vi "Tracking v2.vi"(4 "Offset Home 2 RCM":dbl[](array[numeric])=[0.0, 0.0, 0.0, 0.0], 5 "Trajectory Cluster":T1, 6 "PID Cluster":T4={"L1 to L4 PID Cluster"={"L1 PID Gains"={"Kp"=0.005, "Kd"=0.5, "Ki"=0.0005}, "L2 PID Gains"={"Kp"=0.01, "Kd"=1.0, "Ki"=0.005}, "L3 PID Gains"={"Kp"=0.05, "Kd"=1.0, "Ki"=0.0005}, "L4 PID Gains"={"Kp"=0.1, "Kd"=0.1, "Ki"=0.0005}}, "Stage PID Cluster"={"Stage Z PID"={"Kp"=0.0005, "Kd"=0.001, "Ki"=0.0}, "Stage Y PID"={"Kp"=0.0003, "Kd"=0.01, "Ki"=0.0}, "Stage X PID"={"Kp"=0.0003, "Kd"=0.01, "Ki"=0.0}}, "OCT Z PID Gains"={"Kp"=0.0003, "Kd"=0.0001, "Ki"=0.01}}, 7 "No. Cycles":u8=1, 8 "error in":errorcluster, 10 "Prev Posit Cluster":T3={"Prev L1 to L4 Posit"=[-0.5319, -0.035669172703475985, -2.0566170657346783, 0.9099264705882353], "Prev Stage Posit"=[6.002553885707208, 5.996566124542428, 5.995469940427586], "Prev OCT Z Posit"=-0.0}, 11 "FPGA VI Reference In":refnum<k20>) -> (0 "error out":errorcluster, 2 "Last Posit Cluster":T2={"Last L1 to L4 Posit"=[0.0, 0.0, 0.0, 0.0], "Last Stage Posit"=[6.0, 6.0, 6.0], "Last OCT Z Posit"=0.0}, 3 "FPGA VI Reference Out":refnum<k20>)   [LabVIEW 2016]
uses:
  <vilib>/Platform/TimedLoop/XDataNode/timing_clust.ctl
  <vilib>/Platform/TimedLoop/XDataNode/nitl_modes.ctl
  <vilib>/Platform/TimedLoop/XDataNode/wakeup.ctl
  Global Variables.vi
  <vilib>/platform/TimedLoop/XDataNode/XDataNode.xnode
  <vilib>/Platform/TimedLoop/XDataNode/XDNodeRunTimeDep.lvlib
  Library/KevinLibraryAll/labview/KevLib01.lvlib
panel:
  out "In Servo Loop":bool
  out "Loading Finished":bool
  # "e"
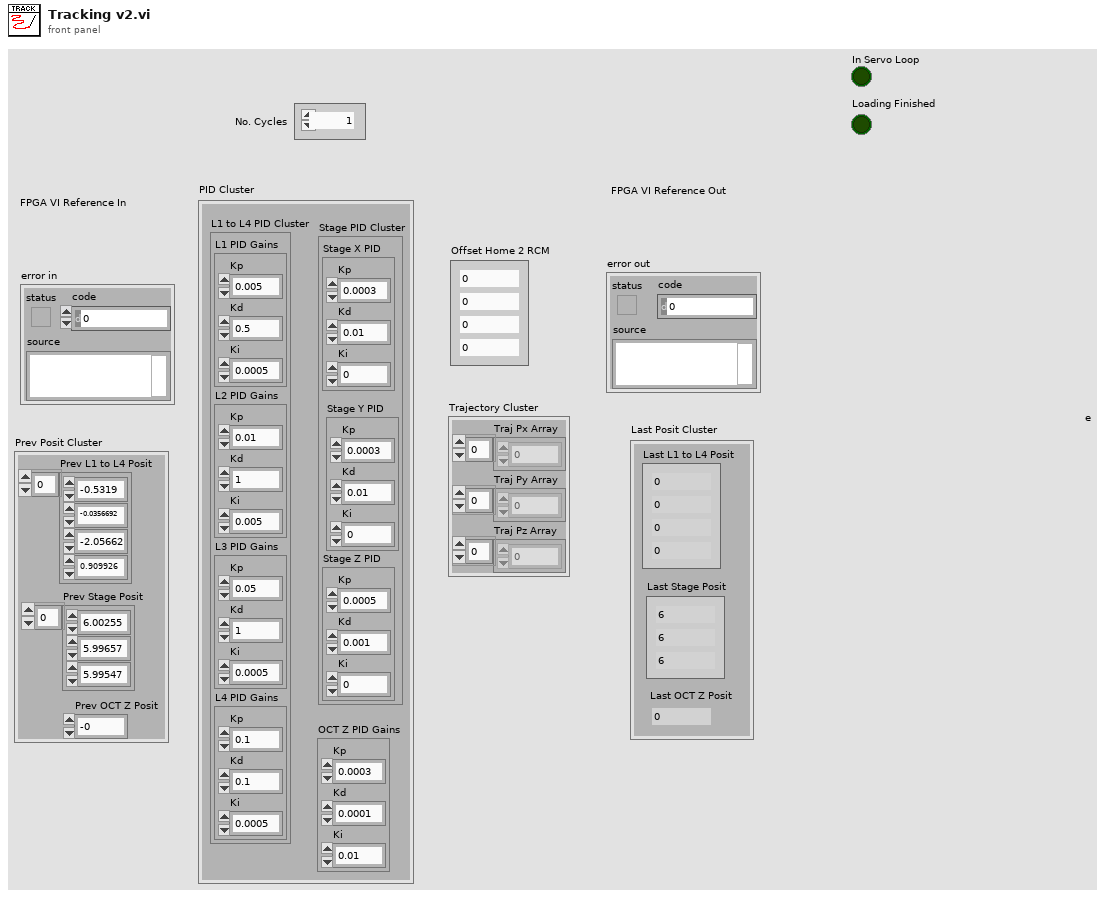
[diagram p1: front panel]
types:
  T1 = cluster{"Traj Px Array":dbl[], "Traj Py Array":dbl[], "Traj Pz Array":dbl[]}
  T2 = cluster{"Last L1 to L4 Posit":dbl[], "Last Stage Posit":dbl[], "Last OCT Z Posit":dbl}
  T3 = cluster{"Prev L1 to L4 Posit":dbl[], "Prev Stage Posit":dbl[], "Prev OCT Z Posit":dbl}
  T4 = cluster{"L1 to L4 PID Cluster":cluster{"L1 PID Gains":cluster{"Kp":dbl, "Kd":dbl, "Ki":dbl}, "L2 PID Gains":cluster{"Kp":dbl, "Kd":dbl, "Ki":dbl}, "L3 PID Gains":cluster{"Kp":dbl, "Kd":dbl, "Ki":dbl}, "L4 PID Gains":cluster{"Kp":dbl, "Kd":dbl, "Ki":dbl}}, "Stage PID Cluster":cluster{"Stage Z PID":cluster{"Kp":dbl, "Kd":dbl, "Ki":dbl}, "Stage Y PID":cluster{"Kp":dbl, "Kd":dbl, "Ki":dbl}, "Stage X PID":cluster{"Kp":dbl, "Kd":dbl, "Ki":dbl}}, "OCT Z PID Gains":cluster{"Kp":dbl, "Kd":dbl, "Ki":dbl}}
  T5 = typedef "XDNodeRunTimeDep.lvlib/timing_clust.ctl" = cluster{"Expected End [f-1]":u64, "Actual End [f-1]":u64, "Finished Late? [f-1]":bool, "Expected End [i-1]":u64, "Actual End [i-1]":u64, "Finished Late? [i-1]":bool, "Expected Start [i]":u64, "Actual Start [i]":u64, "Expected Start [f]":u64, "Actual Start [f]":u64, "Source Name":string, "Structure Name":string, "Period":i64, "Deadline":i64, "Offset":i64, "Start":i64, "Priority":i32, "Timeout":i32, "Mode":T6, "Wakeup Reason":T7, "Error":errorcluster, "Source Type":string, "Secondary Source Type":string, "Global End Time":u64, "Global Start Time":u64, "Frame Duration":u64, "Iteration Duration":u64, "Assigned CPU":i32, "I/O Scan Engine Mode":u32}
  T6 = typedef "XDNodeRunTimeDep.lvlib/nitl_modes.ctl" = enum32{"No Change", "Process missed periods, maintain original phase", "Discard missed periods, maintain original phase", "Process missed periods, ignore original phase", "Discard missed periods, ignore original phase"}
  T7 = typedef "XDNodeRunTimeDep.lvlib/wakeup.ctl" = enum32{"Normal", "Aborted", "Asynchronous wakeup", "Timing source error", "Timed loop error", "Timeout"}
  T8 = cluster{"L1 PID Gains":cluster{"Kp":dbl, "Kd":dbl, "Ki":dbl}, "L2 PID Gains":cluster{"Kp":dbl, "Kd":dbl, "Ki":dbl}, "L3 PID Gains":cluster{"Kp":dbl, "Kd":dbl, "Ki":dbl}, "L4 PID Gains":cluster{"Kp":dbl, "Kd":dbl, "Ki":dbl}}
  T9 = cluster{"Stage Z PID":cluster{"Kp":dbl, "Kd":dbl, "Ki":dbl}, "Stage Y PID":cluster{"Kp":dbl, "Kd":dbl, "Ki":dbl}, "Stage X PID":cluster{"Kp":dbl, "Kd":dbl, "Ki":dbl}}
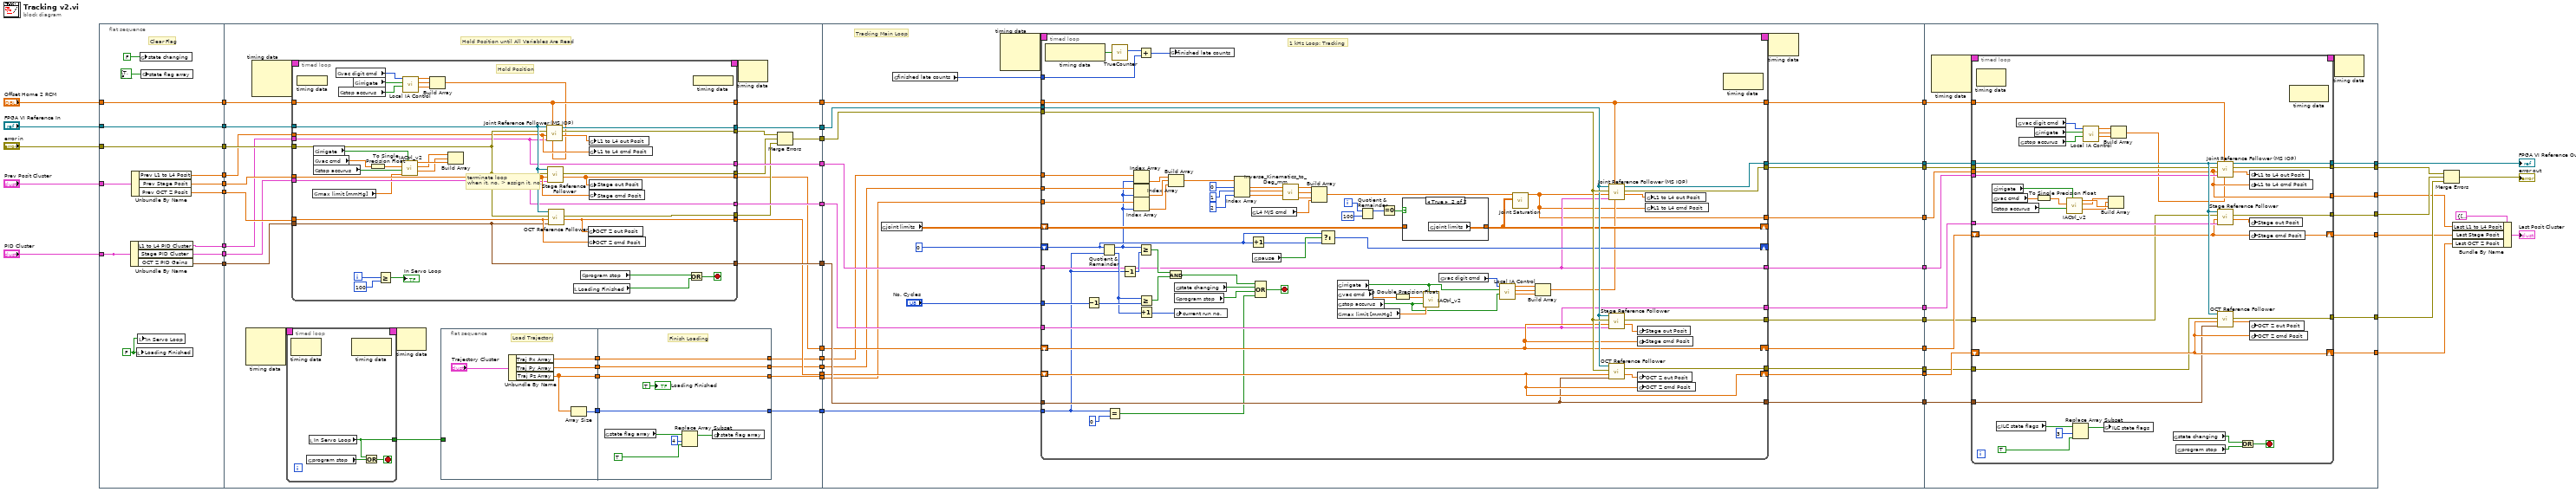
[diagram p0: block diagram]
diagram:
  n1 = flat-sequence {
    tunnel: [w59] -> w47
    tunnel: "FPGA VI Reference In" -> [w59]
    tunnel: "error in" -> [w58]
    tunnel: [w58] -> w44
    tunnel: "Prev Posit Cluster" -> [w57]
    tunnel: [w56] -> _
    tunnel: "PID Cluster" -> [w56]
    tunnel: [w55] -> w41
    tunnel: [w54] -> w40
    tunnel: [w53] -> w39
    tunnel: [w52] -> w38
    tunnel: [w51] -> w37
    tunnel: "Offset Home 2 RCM" -> [w51]
    tunnel: [w50] -> w32
    tunnel: [w48] -> w23
    tunnel: w47 -> [w94]
    tunnel: w44 -> [w93]
    tunnel: w41 -> [w92]
    tunnel: w40 -> [w91]
    tunnel: w39 -> [w90]
    tunnel: w38 -> [w89]
    tunnel: w37 -> [w88]
    tunnel: [w87] -> w35
    tunnel: [w86] -> w34
    tunnel: [w85] -> w33
    tunnel: w32 -> [w84]
    tunnel: [w83] -> w31
    tunnel: [w82] -> w30
    tunnel: [w81] -> w29
    tunnel: w23 -> [w80]
    tunnel: [w74] -> w22
    tunnel: [w73] -> w21
    tunnel: [w66] -> w20
    tunnel: [w65] -> w19
    tunnel: [w64] -> w18
    tunnel: [w62] -> w17
    tunnel: w35 -> [w183]
    tunnel: w34 -> [w168]
    tunnel: w33 -> [w182]
    tunnel: w31 -> [w180]
    tunnel: w30 -> [w179]
    tunnel: w29 -> [w178]
    tunnel: w22 -> [w170]
    tunnel: w21 -> [w169]
    tunnel: w20 -> [w167]
    tunnel: w19 -> [w166]
    tunnel: w18 -> [w165]
    tunnel: w17 -> [w157]
    tunnel: [w177] -> w16
    tunnel: [w176] -> w15
    tunnel: [w175] -> w14
    tunnel: [w174] -> w13
    tunnel: [w173] -> w12
    tunnel: [w172] -> w11
    tunnel: [w171] -> w10
    tunnel: [w161] -> w9
    tunnel: [w160] -> w8
    tunnel: [w159] -> w7
    tunnel: [w158] -> w6
    tunnel: [w275] -> w24
    tunnel: [w281] -> w2
    tunnel: [w276] -> w3
    tunnel: [w268] -> w5
    tunnel: [w269] -> w25
    tunnel: w16 -> [w273]
    tunnel: w15 -> [w272]
    tunnel: w14 -> [w277]
    tunnel: w13 -> [w279]
    tunnel: w12 -> [w282]
    tunnel: w11 -> [w278]
    tunnel: w10 -> [w280]
    tunnel: w9 -> [w283]
    tunnel: w8 -> [w274]
    tunnel: w7 -> [w271]
    tunnel: w6 -> [w270]
    tunnel: [w267] -> w4
    tunnel: [w266] -> w1
    frame #0 {
      w49 = FALSE ("Loading Finished")
      # "Clear Flag"
      n2 = Unbundle By Name(w56) -> ("L1 to L4 PID Cluster"=w52:T8, "Stage PID Cluster"=w50:T9, "OCT Z PID Gains"=w55:cluster{"Kp":dbl, "Kd":dbl, "Ki":dbl})
      n3 = Unbundle By Name(w57) -> ("Prev L1 to L4 Posit"=w48:dbl[], "Prev Stage Posit"=w54:dbl[], "Prev OCT Z Posit"=w53:dbl)
      n4 = local write "Loading Finished"(w49) -> ()
      n5 = local write "In Servo Loop"(w49) -> ()
      n6 = global write "Global Variables.vi" "state changing"(FALSE ("state changing")) -> ()
      n7 = global write "Global Variables.vi" "state flag array"(bool[] [TRUE, FALSE, FALSE, FALSE, FALSE, FALSE, FALSE, FALSE, FALSE] ("state flag array")) -> ()
    }
    frame #1 {
      # "terminate loop\nwhen it. no. > assign it. no."
      # "Hold Position until All Variables Are Read"
      n8 = node-c288() -> (w72:T5)  [unwired: 3 in]
      n9 = node-c288() -> (w79:T5)  [unwired: 3 in]
      n10 = timed-loop {
        timing: w72 -> [_]
        timing-out: [_] -> w71
        tunnel: [w109] -> w70
        stop <- w111 stop-if-true
        n11 = node-c288() -> ()  [unwired: 1 in, 1 out]
        n12 = global read "Global Variables.vi" "program stop"() -> (w110:bool)
        n13 = local read "In Servo Loop"() -> (w109:bool)
        n14 = node-c288() -> ()  [unwired: 1 in, 1 out]
        n15 = Or(x=w109, y=w110) -> (x .or. y?=w111:bool)
      }
      n16 = timed-loop {
        timing: w79 -> [_]
        timing-out: [_] -> w78
        tunnel: [w148] -> w74
        tunnel: [w147] -> w73
        tunnel: [w146] -> w87
        tunnel: [w145] -> w77
        tunnel: [w144] -> w76
        tunnel: [w143] -> w75
        tunnel: w94 -> [w142]
        tunnel: w93 -> [w141]
        tunnel: w92 -> [w136]
        tunnel: w80 -> [w139]
        tunnel: w91 -> [w140]
        tunnel: w90 -> [w138]
        tunnel: w89 -> [w134]
        tunnel: w88 -> [w137]
        tunnel: [w137] -> w86
        tunnel: w84 -> [w135]
        tunnel: [w136] -> w81
        tunnel: [w135] -> w82
        tunnel: [w134] -> w83
        i -> [w133]
        stop <- w152 stop-if-true
        # "Hold Position"
        n17 = node-c288 ("Output Node")() -> ()  [unwired: 1 in]
        n18 = global read "Global Variables.vi" "max limit [mmHg]"() -> (w123:dbl)
        n19 = global read "Global Variables.vi" "irrigate"() -> (w129:bool)
        n20 = global read "Global Variables.vi" "vac cmd"() -> (w126:sgl)
        n21 = global read "Global Variables.vi" "stop accurus"() -> (w125:bool)
        n22 = global read "Global Variables.vi" "vac digit cmd"() -> (w121:i8)
        n23 = global read "Global Variables.vi" "stop accurus"() -> (w120:bool)
        n24 = global read "Global Variables.vi" "irrigate"() -> (w122:bool)
        n25 = To Single Precision Float(number=w126) -> (single precision float=w127:sgl)
        n26 = Greater Or Equal?(x=w133, y=100) -> (x >= y?=→"In Servo Loop":bool)
        n27 = call "IACtrl_v2.vi"("Irrigate?"=w129, "Max Limit [mmHg]"=w123, "E-Stop Vacuum"=w125, "Vacuum Force [mmHg]"=w127) -> ("Accurus ChB Vout"=w124:dbl, "Accurus ChA Vout"=w128:dbl, "Accurus Engaged Vout"=w130:dbl)  [unwired: 4 in, 1 out]
        n28 = call "Local IA Control.vi"("E-Stop Vacuum"=w120, "Irrigate?"=w122, "8bit integer"=w121) -> ("Accurus Engaged Vout"=w117:dbl, "Accurus ChB Vout"=w118:dbl, "Accurus ChA Vout"=w119:dbl)  [unwired: 6 in]
        n29 = Build Array(w119, w118, w117) -> (w116:dbl[])
        n30 = Build Array(w128, w124, w130) -> ()  [unwired: 1 out]
        n31 = call "Joint Reference Follower (MS IOP).vi"("Acc Ctrl Array"=w116, "Offset Home2RCM [deg/mm]"=w137, "PID Ctrl Cluster"=w134, "Ref Array [deg/mm]"=w139, "error in"=w141, "FPGA VI Reference In"=w142) -> ("Output Posit Array [deg/mm]"=w149:dbl[], "error out"=w145:errorcluster, "FPGA VI Reference Out"=w146:refnum<k20>)  [unwired: 3 in]
        n32 = call "Stage Reference Follower.vi"("Stage PID Cluster"=w135, "Stage cmd Posit [mm]"=w140, "error in"=w141, "FPGA VI Reference In"=w142) -> ("Stage out Posit [mm]"=w148:dbl[], "error out"=w144:errorcluster)  [unwired: 5 in, 1 out]
        n33 = call "OCT Reference Follower.vi"("OCT Z PID Gains"=w136, "OCT  Z cmd Posit [mm]"=w138, "error in"=w141, "FPGA VI Reference In"=w142) -> ("OCT  Z out Posit [mm]"=w147:dbl, "error out"=w143:errorcluster)  [unwired: 5 in, 1 out]
        n34 = local read "Loading Finished"() -> (w151:bool)
        n35 = global read "Global Variables.vi" "program stop"() -> (w150:bool)
        n36 = global write "Global Variables.vi" "OCT Z out Posit"(w147) -> ()
        n37 = global write "Global Variables.vi" "OCT Z cmd Posit"(w138) -> ()
        n38 = global write "Global Variables.vi" "L1 to L4 out Posit"(w149) -> ()
        n39 = global write "Global Variables.vi" "L1 to L4 cmd Posit"(w139) -> ()
        n40 = global write "Global Variables.vi" "Stage out Posit"(w148) -> ()
        n41 = global write "Global Variables.vi" "Stage cmd Posit"(w140) -> ()
        n42 = Or(x=w150, y=w151) -> (x .or. y?=w152:bool)
        n43 = node-c288() -> ()  [unwired: 1 out]
      }
      n44 = node-c288(w71) -> ()  [unwired: 1 out]
      n45 = flat-sequence {
        tunnel: w70 -> [_]
        tunnel: [w98] -> w69
        tunnel: [w97] -> w68
        tunnel: [w96] -> w67
        tunnel: [w95] -> w63
        tunnel: w69 -> [w105]
        tunnel: w68 -> [w106]
        tunnel: w67 -> [w107]
        tunnel: [w107] -> w66
        tunnel: [w106] -> w65
        tunnel: [w105] -> w64
        tunnel: w63 -> [w104]
        tunnel: [w104] -> w62
        frame #0 {
          # "Load Trajectory"
          n46 = Unbundle By Name("Trajectory Cluster") -> ("Traj Px Array"=w96:dbl[], "Traj Py Array"=w97:dbl[], "Traj Pz Array"=w98:dbl[])
          n47 = Array Size(array=w98) -> (size(s)=w95:i32)
        }
        frame #1 {
          # "Finish Loading"
          n48 = global read "Global Variables.vi" "state flag array"() -> (w101:bool[])
          n49 = Replace Array Subset(array=w101, new element=TRUE ("new element/subarray"), index=4) -> (w100:bool[])
          n50 = global write "Global Variables.vi" "state flag array"(w100) -> ()
          "Loading Finished" <- TRUE ("Loading Finished")
        }
      }
      n51 = node-c288(w78) -> ()  [unwired: 1 out]
      n52 = Merge Errors(w77, w76, w75) -> (w85:errorcluster)
    }
    frame #2 {
      # "Tracking Main Loop"
      n53 = global read "Global Variables.vi" "joint limits"() -> (w162:dbl[][])
      n54 = global read "Global Variables.vi" "finished late counts"() -> (w181:u16)
      n55 = node-c288() -> (w185:T5)  [unwired: 3 in]
      n56 = timed-loop {
        timing: w185 -> [_]
        timing-out: [_] -> w184
        tunnel: w167 -> [w258]
        tunnel: w166 -> [w257]
        tunnel: w165 -> [w241]
        tunnel: w183 -> [w253]
        tunnel: w168 -> [w202]
        tunnel: w182 -> [w254]
        tunnel: [w255] -> w177
        tunnel: w180 -> [w199]
        tunnel: w181 -> [w249]
        tunnel: w179 -> [w201]
        tunnel: w178 -> [w200]
        shift-right: [w204] -> w172
        shift-left: w170 -> [w204]
        shift-right: [w203] -> w171
        shift-left: w169 -> [w203]
        tunnel: [w246] -> w175
        tunnel: [w245] -> w174
        tunnel: [w244] -> w176
        tunnel: [w194] -> w173
        tunnel: "No. Cycles" -> [w217]
        shift-right: [w215] -> _
        shift-left: 0 ("No. Cycles") -> [w198]
        tunnel: w157 -> [w197]
        shift-right: [w210] -> _
        shift-left: w162 -> [w209]
        tunnel: [w202] -> w161
        tunnel: [w201] -> w158
        tunnel: [w200] -> w160
        tunnel: [w199] -> w159
        i -> [w214]
        stop <- w222 stop-if-true
        # "Hold Position if not Engaged"
        # "1 kHz Loop: Tracking"
        n57 = node-c288() -> (w252:bool)  [unwired: 1 in]
        n58 = Decrement(x=w217) -> (x-1=w228:u8)
        n59 = Quotient & Remainder(x=w198, y=w197) -> (x-y*floor(x/y)=w192:i32, floor(x/y)=w216:i32)
        n60 = Equal?(x=w197, y=0) -> (x = y?=w195:bool)
        n61 = call "TrueCounter.vi"("True?"=w252) -> ("True Count"=w250:u16)  [unwired: 10 in]
        n62 = Decrement(x=w197) -> (x-1=w229:i32)
        n63 = Index Array(array=w258, index=w192) -> (element=w233:dbl)
        n64 = Index Array(array=w257, index=w192) -> (element=w232:dbl)
        n65 = Index Array(array=w241, index=w192) -> (element=w231:dbl)
        n66 = Add(x=w250, y=w249) -> (x+y=w251:u16)
        n67 = Greater Or Equal?(x=w192, y=w229) -> (x >= y?=w227:bool)
        n68 = Greater Or Equal?(x=w216, y=w228) -> (x >= y?=w226:bool)
        n69 = Increment(x=w216) -> (x+1=w218:i32)
        n70 = And(x=w227, y=w226) -> (x .and. y?=w225:bool)
        n71 = Build Array(w233, w232, w231) -> (w230:dbl[])
        n72 = global write "Global Variables.vi" "finished late counts"(w251) -> ()
        n73 = global read "Global Variables.vi" "state changing"() -> (w224:bool)
        n74 = global read "Global Variables.vi" "program stop"() -> (w223:bool)
        n75 = global write "Global Variables.vi" "current run no."(w218) -> ()
        n76 = Index Array(array=w230, index #1=0 ("index"), index #2=1 ("index"), index #3=2 ("index")) -> (element #1=w236:dbl, element #2=w235:dbl, element #3=w234:dbl)
        n77 = Increment(x=w198) -> (x+1=w219:i32)
        n78 = global read "Global Variables.vi" "L4 M/S cmd"() -> (w221:dbl)
        n79 = global read "Global Variables.vi" "pause"() -> (w220:bool)
        n80 = Compound Arithmetic op=OR(w225, w224, w223, w195) -> (w222:bool)
        n81 = call "Inverse_Kinematics_to_Deg_mm.vi"("pz"=w234, "py"=w235, "px"=w236) -> ("L3 [mm]"=w242:dbl, "L2 [deg]"=w243:dbl, "L1 [deg]"=w256:dbl)
        n82 = Build Array(w256, w243, w242, w221) -> (w240:dbl[])
        n83 = Select(t=w198, s=w220, f=w219) -> (s? t:f=w215:i32)
        n84 = global read "Global Variables.vi" "irrigate"() -> (w189:bool)
        n85 = global read "Global Variables.vi" "vac cmd"() -> (w208:sgl)
        n86 = global read "Global Variables.vi" "stop accurus"() -> (w188:bool)
        n87 = global read "Global Variables.vi" "max limit [mmHg]"() -> (w206:dbl)
        n88 = Quotient & Remainder(x=w214, y=100) -> (x-y*floor(x/y)=w212:i32)  [unwired: 1 out]
        n89 = Equal To 0?(x=w212) -> (x = 0?=w211:bool)
        n90 = To Double Precision Float(number=w208) -> (double precision float=w207:dbl)
        n91 = case shown="True" w211 {
          tunnel: [w259 w260] -> w210
          tunnel: w209 -> [w259 _]
          frame False {
          }
          frame True {
            n92 = global read "Global Variables.vi" "joint limits"() -> (w260:dbl[][])
          }
        }
        n93 = call "IACtrl_v2.vi"("Irrigate?"=w189, "Max Limit [mmHg]"=w206, "E-Stop Vacuum"=w188, "Vacuum Force [mmHg]"=w207) -> ()  [unwired: 4 in, 4 out]
        n94 = global read "Global Variables.vi" "vac digit cmd"() -> (w190:i8)
        n95 = call "Local IA Control.vi"("E-Stop Vacuum"=w188, "Irrigate?"=w189, "8bit integer"=w190) -> ("Accurus Engaged Vout"=w186:dbl, "Accurus ChB Vout"=w187:dbl, "Accurus ChA Vout"=w191:dbl)  [unwired: 6 in]
        n96 = call "Joint Saturation.vi"("Joint Bounds [Deg/mm]"=w210, "Ref Array [Deg/mm]"=w240) -> ("Sat Ref Array [Deg/mm]"=w194:dbl[])  [unwired: 9 in]
        n97 = Build Array(w191, w187, w186) -> (w205:dbl[])
        n98 = call "Joint Reference Follower (MS IOP).vi"("Acc Ctrl Array"=w205, "Offset Home2RCM [deg/mm]"=w202, "PID Ctrl Cluster"=w199, "Ref Array [deg/mm]"=w194, "error in"=w254, "FPGA VI Reference In"=w253) -> ("Output Posit Array [deg/mm]"=w193:dbl[], "error out"=w244:errorcluster, "FPGA VI Reference Out"=w255:refnum<k20>)  [unwired: 3 in]
        n99 = call "Stage Reference Follower.vi"("Stage PID Cluster"=w201, "Stage cmd Posit [mm]"=w204, "error in"=w254, "FPGA VI Reference In"=w253) -> ("Stage out Posit [mm]"=w248:dbl[], "error out"=w246:errorcluster)  [unwired: 5 in, 1 out]
        n100 = call "OCT Reference Follower.vi"("OCT Z PID Gains"=w200, "OCT  Z cmd Posit [mm]"=w203, "error in"=w254, "FPGA VI Reference In"=w253) -> ("OCT  Z out Posit [mm]"=w247:dbl, "error out"=w245:errorcluster)  [unwired: 5 in, 1 out]
        n101 = global write "Global Variables.vi" "Stage out Posit"(w248) -> ()
        n102 = global write "Global Variables.vi" "Stage cmd Posit"(w204) -> ()
        n103 = global write "Global Variables.vi" "OCT Z out Posit"(w247) -> ()
        n104 = global write "Global Variables.vi" "OCT Z cmd Posit"(w203) -> ()
        n105 = global write "Global Variables.vi" "L1 to L4 out Posit"(w193) -> ()
        n106 = global write "Global Variables.vi" "L1 to L4 cmd Posit"(w194) -> ()
        n107 = node-c288() -> ()  [unwired: 1 in, 1 out]
      }
      n108 = node-c288(w184) -> ()  [unwired: 1 out]
    }
    frame #3 {
      n109 = node-c288() -> (w285:T5)  [unwired: 3 in]
      n110 = timed-loop {
        timing: w285 -> [_]
        timing-out: [_] -> w284
        tunnel: w273 -> [w321]
        tunnel: w271 -> [w320]
        tunnel: w270 -> [w319]
        tunnel: w279 -> [w306]
        tunnel: w282 -> [w310]
        tunnel: w283 -> [w318]
        tunnel: [w317] -> w269
        tunnel: [w316] -> w268
        tunnel: [w310] -> w281
        tunnel: [w312] -> w267
        tunnel: [w311] -> w276
        shift-right: [w309] -> w266
        shift-left: w278 -> [w309]
        shift-right: [w308] -> w275
        shift-left: w280 -> [w308]
        tunnel: w277 -> [w307]
        tunnel: w274 -> [w305]
        tunnel: w272 -> [w304]
        stop <- w324 stop-if-true
        n111 = node-c288() -> ()  [unwired: 1 in, 1 out]
        n112 = global read "Global Variables.vi" "irrigate"() -> (w302:bool)
        n113 = global read "Global Variables.vi" "vac cmd"() -> (w299:sgl)
        n114 = global read "Global Variables.vi" "stop accurus"() -> (w298:bool)
        n115 = global read "Global Variables.vi" "ILC state flags"() -> (w295:bool[])
        n116 = global read "Global Variables.vi" "vac digit cmd"() -> (w291:i8)
        n117 = global read "Global Variables.vi" "stop accurus"() -> (w290:bool)
        n118 = global read "Global Variables.vi" "irrigate"() -> (w292:bool)
        n119 = To Single Precision Float(number=w299) -> (single precision float=w300:sgl)
        n120 = call "IACtrl_v2.vi"("Irrigate?"=w302, "E-Stop Vacuum"=w298, "Vacuum Force [mmHg]"=w300) -> ("Accurus ChB Vout"=w297:dbl, "Accurus ChA Vout"=w301:dbl, "Accurus Engaged Vout"=w303:dbl)  [unwired: 5 in, 1 out]
        n121 = Replace Array Subset(array=w295, new element=TRUE ("new element/subarray"), index=3) -> (w294:bool[])
        n122 = call "Local IA Control.vi"("E-Stop Vacuum"=w290, "Irrigate?"=w292, "8bit integer"=w291) -> ("Accurus Engaged Vout"=w287:dbl, "Accurus ChB Vout"=w288:dbl, "Accurus ChA Vout"=w289:dbl)  [unwired: 6 in]
        n123 = global write "Global Variables.vi" "ILC state flags"(w294) -> ()
        n124 = Build Array(w301, w297, w303) -> ()  [unwired: 1 out]
        n125 = Build Array(w289, w288, w287) -> (w286:dbl[])
        n126 = global read "Global Variables.vi" "state changing"() -> (w323:bool)
        n127 = global read "Global Variables.vi" "program stop"() -> (w322:bool)
        n128 = call "Joint Reference Follower (MS IOP).vi"("Acc Ctrl Array"=w286, "Offset Home2RCM [deg/mm]"=w318, "PID Ctrl Cluster"=w320, "Ref Array [deg/mm]"=w310, "error in"=w304, "FPGA VI Reference In"=w321) -> ("Output Posit Array [deg/mm]"=w315:dbl[], "error out"=w316:errorcluster, "FPGA VI Reference Out"=w317:refnum<k20>)  [unwired: 3 in]
        n129 = call "Stage Reference Follower.vi"("Stage PID Cluster"=w319, "Stage cmd Posit [mm]"=w309, "error in"=w307, "FPGA VI Reference In"=w321) -> ("Stage out Posit [mm]"=w314:dbl[], "error out"=w312:errorcluster)  [unwired: 5 in, 1 out]
        n130 = call "OCT Reference Follower.vi"("OCT Z PID Gains"=w305, "OCT  Z cmd Posit [mm]"=w308, "error in"=w306, "FPGA VI Reference In"=w321) -> ("OCT  Z out Posit [mm]"=w313:dbl, "error out"=w311:errorcluster)  [unwired: 5 in, 1 out]
        n131 = Or(x=w323, y=w322) -> (x .or. y?=w324:bool)
        n132 = global write "Global Variables.vi" "L1 to L4 out Posit"(w315) -> ()
        n133 = global write "Global Variables.vi" "L1 to L4 cmd Posit"(w310) -> ()
        n134 = global write "Global Variables.vi" "Stage out Posit"(w314) -> ()
        n135 = global write "Global Variables.vi" "Stage cmd Posit"(w309) -> ()
        n136 = global write "Global Variables.vi" "OCT Z out Posit"(w313) -> ()
        n137 = global write "Global Variables.vi" "OCT Z cmd Posit"(w308) -> ()
        n138 = node-c288() -> ()  [unwired: 1 in, 1 out]
      }
      n139 = node-c288(w284) -> ()  [unwired: 1 out]
    }
  }
  n140 = Merge Errors(w5, w4, w3) -> (→"error out":errorcluster)
  n141 = Bundle By Name(cluster=T2 {"Last L1 to L4 Posit"=[0.0, 0.0, 0.0, 0.0], "Last Stage Posit"=[6.0, 6.0, 6.0], "Last OCT Z Posit"=0.0} ("Last Posit Cluster 2"), "Last L1 to L4 Posit"=w2, "Last Stage Posit"=w1, "Last OCT Z Posit"=w24) -> (→"Last Posit Cluster":T2)
  "FPGA VI Reference Out" <- w25
